vi "Write_Speaker.vi"(5 "Characteristic UUID":string, 6 "Connection Status":T1={"MAC Address"="", "cnx handle"=0, "cnx flags"=0, "Address Type"=125, "Connection Interval (ms)"=125, "Timeout(ms)"=125, "Latency"=0, "bonding handle"=0} {"Address Type" items=["Public", "Random"]}, 7 "Service UUID":string, 8 "error in (no error)":errorcluster, 9 "Sample":u8, 10 "Handle table":string[][](array[string]), 11 "COM Bluegiga in":refnum<visa-resource-name>) -> (0 "error out":errorcluster, 3 "COM Bluegiga out":refnum<visa-resource-name>)   [LabVIEW 2020]
uses:
  <vilib>/BLE/type_def/connection_status_bundle.ctl
  <vilib>/BLE/type_def/address_type.ctl
  <vilib>/BLE/ble_functions/ble_write_by_service_characteristic_uint8array.vi
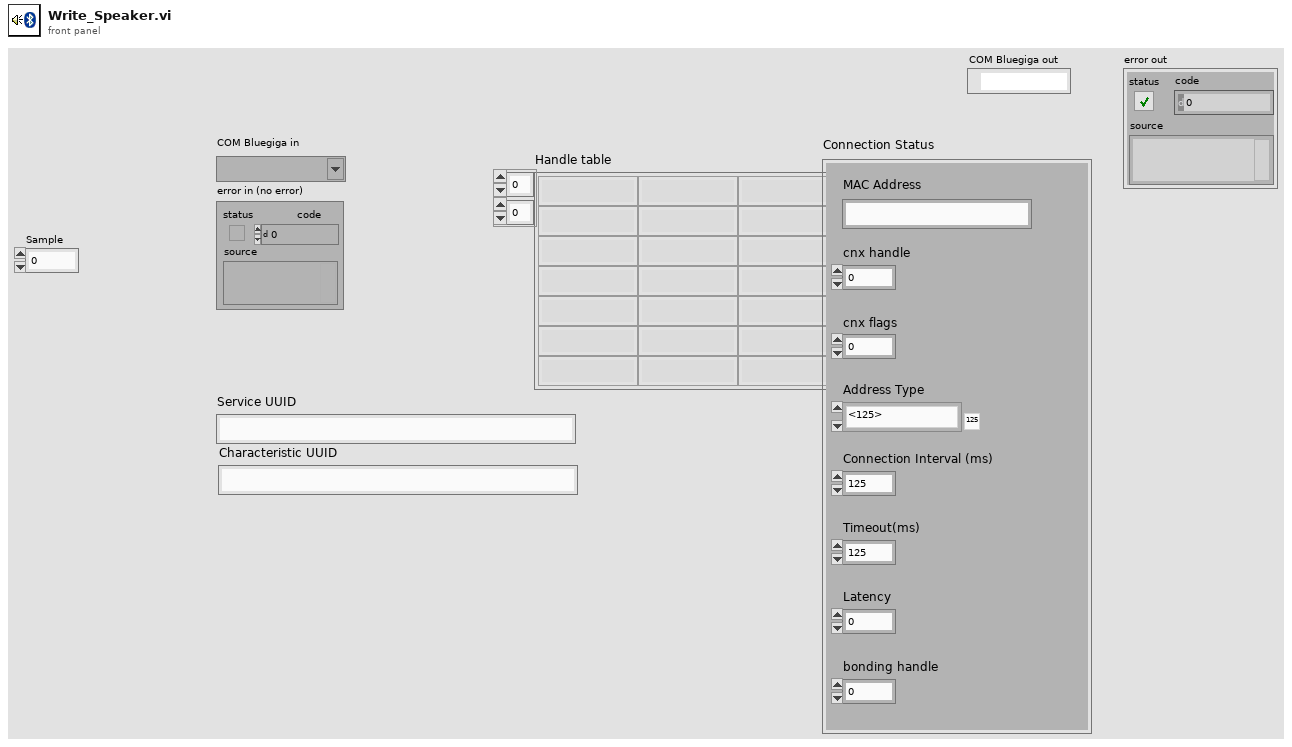
[diagram p1: front panel]
types:
  T1 = typedef "connection_status_bundle.ctl" = cluster{"MAC Address":string, "cnx handle":u8, "cnx flags":u8, "Address Type":T2, "Connection Interval (ms)":u16, "Timeout(ms)":u16, "Latency":u16, "bonding handle":u8}
  T2 = typedef "address_type.ctl" = u8
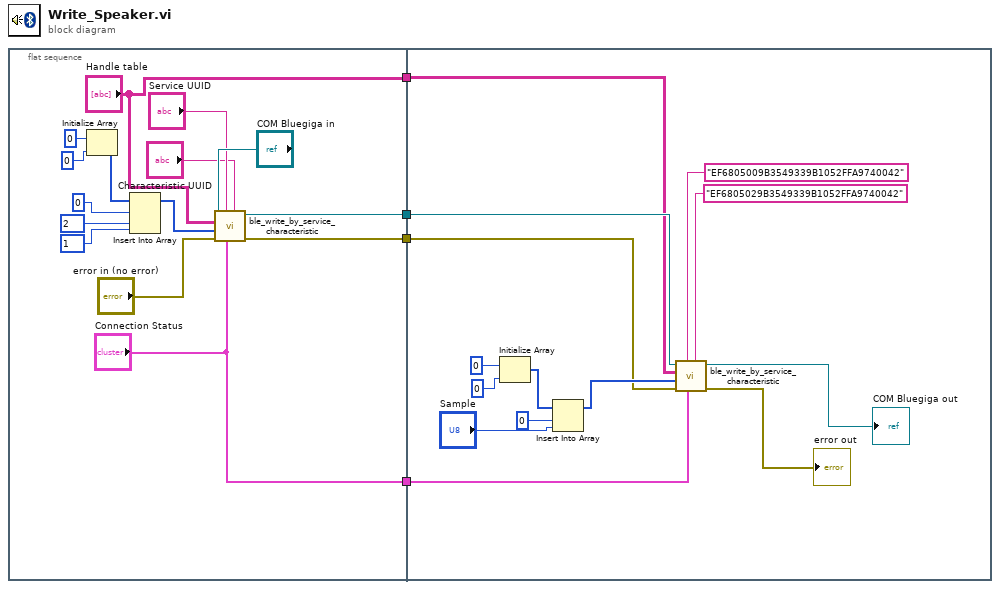
[diagram p0: block diagram]
diagram:
  n1 = flat-sequence {
    tunnel: [w12] -> w4
    tunnel: [w11] -> w3
    tunnel: ["Connection Status"] -> w2
    tunnel: ["Handle table"] -> w1
    tunnel: w4 -> [w25]
    tunnel: w3 -> [w24]
    tunnel: w2 -> [w21]
    tunnel: w1 -> [w20]
    frame #0 {
      n2 = Initialize Array(u8 0 ("element"), 0 ("dimension size")) -> (w13:u8[])
      n3 = Insert Into Array(array=w13, index=0, new element #1=u8 2 ("new element/subarray"), new element #2=u8 1 ("new element/subarray")) -> (w16:u8[])
      n4 = call-poly <vilib>:"ble_write_by_service_characteristic.vi"("Characteristic UUID"="Characteristic UUID", "Connection Status"="Connection Status", "Service UUID"="Service UUID", "error in (no error)"="error in (no error)", "data"=w16, "Handle table"="Handle table", "COM Bluegiga in"="COM Bluegiga in") -> ("error out"=w11:errorcluster, "COM Bluegiga out"=w12:refnum<visa-resource-name>)  [unwired: 3 in]
    }
    frame #1 {
      n5 = Initialize Array(u8 0 ("element"), 0 ("dimension size")) -> (w30:u8[])
      n6 = Insert Into Array(array=w30, index=0, new element="Sample") -> (w26:u8[])
      n7 = call-poly <vilib>:"ble_write_by_service_characteristic.vi"("Characteristic UUID"="EF6805029B3549339B1052FFA9740042", "Connection Status"=w21, "Service UUID"="EF6805009B3549339B1052FFA9740042", "error in (no error)"=w24, "data"=w26, "Handle table"=w20, "COM Bluegiga in"=w25) -> ("error out"=→"error out":errorcluster, "COM Bluegiga out"=→"COM Bluegiga out":refnum<visa-resource-name>)  [unwired: 3 in]
    }
  }
